vi "Delete Curve.vi"(8 "error in (no error)":errorcluster, 10 "Curve to Erase (21)":i32=21 min=21 max=59 step=1, 11 "VISA resource name":refnum<visa-resource-name>) -> (0 "error out":errorcluster, 3 "VISA resource name out":refnum<visa-resource-name>)   [LabVIEW 2015, in "Lake Shore 372.lvlib"]
doc: "Deletes the selected user curve."
uses:
  <instrlib>/Lake Shore 372/Lake Shore 372.lvlib
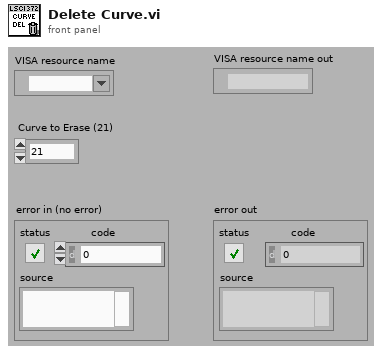
[diagram p1: front panel]
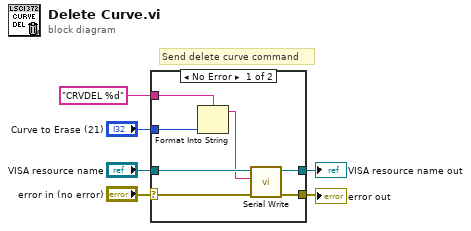
[diagram p0: block diagram]
diagram:
  # "Send delete curve command"
  n1 = case shown="No Error" "error in (no error)" {
    selector: "error in (no error)" -> [w7 w14]
    tunnel: [w13 w14] -> w6
    tunnel: [w12 w15] -> w5
    tunnel: "VISA resource name" -> [w11 w15]
    tunnel: "CRVDEL %d" -> [w10 _]
    tunnel: "Curve to Erase (21)" -> [w9 _]
    frame No Error {
      n2 = Format Into String(format string=w10, w9) -> (resulting string=w8:string)  [unwired: 2 in, 1 out]
      n3 = call <instrlib>:"Serial Write.vi"("error in (no error)"=w7, "Write Buffer (\"\")"=w8, "VISA resource name"=w11) -> ("error out"=w13:errorcluster, "VISA resource name out"=w12:refnum<visa-resource-name>)  [unwired: 6 in, 1 out]
    }
    frame Error {
    }
  }
  "error out" <- w6
  "VISA resource name out" <- w5
